vi "Error Check Columns.vi"(8 "error in (no error)":errorcluster, 10 "Columns in":refnum<class "Column.lvclass">[](array[class]), 11 "Slave_Pulseblaster in":refnum<class "Slave_Pulseblaster.lvclass">) -> (0 "error out":errorcluster, 2 "Columns OK":bool, 3 "Slave_Pulseblaster out":refnum<class "Slave_Pulseblaster.lvclass">)   [LabVIEW 2013, in "Slave_Pulseblaster.lvclass"]
uses:
  Slave_Pulseblaster.lvclass
  ColumnVIs/Column/Column.lvclass
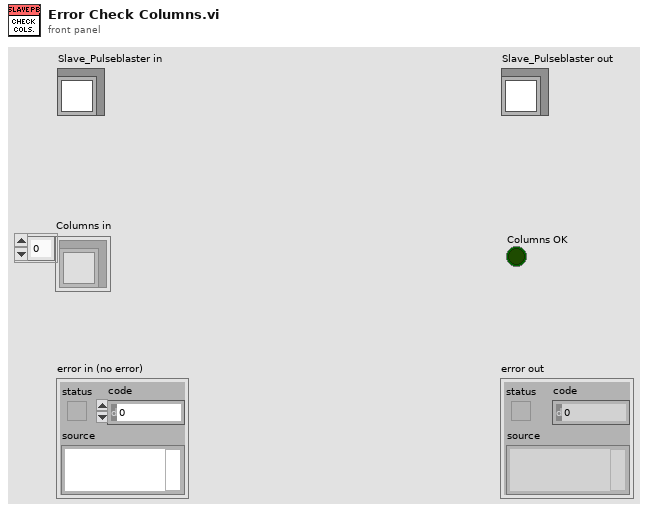
[diagram p1: front panel]
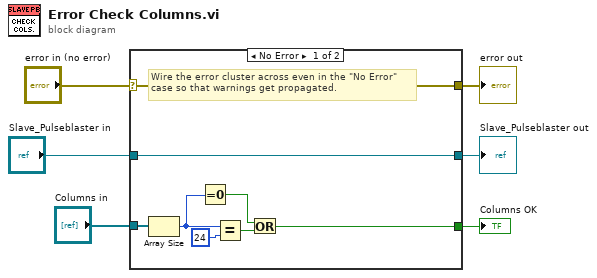
[diagram p0: block diagram]
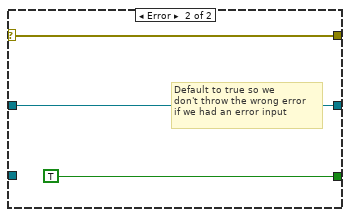
[diagram p2: hidden frame]
diagram:
  n1 = case shown="No Error" "error in (no error)" {
    selector: "error in (no error)" -> [w13 w17]
    tunnel: [w13 w17] -> w5
    tunnel: [w14 w16] -> w3
    tunnel: "Slave_Pulseblaster in" -> [w14 w16]
    tunnel: "Columns in" -> [w8 _]
    tunnel: [w7 TRUE] -> w1
    frame No Error {
      # "Wire the error cluster across even in the \"No Error\"\ncase so that warnings get propagated."
      n2 = Array Size(array=w8) -> (size(s)=w12:i32)
      n3 = Equal To 0?(x=w12) -> (x = 0?=w11:bool)
      n4 = Equal?(x=w12, y=24) -> (x = y?=w10:bool)
      n5 = Or(x=w11, y=w10) -> (x .or. y?=w7:bool)
    }
    frame Error {
      # "Default to true so we\ndon't throw the wrong error\nif we had an error input"
    }
  }
  "error out" <- w5
  "Slave_Pulseblaster out" <- w3
  "Columns OK" <- w1
